vi "Average_center.vi"() -> ()   [LabVIEW 2012]
uses:
  <vilib>/Utility/file.llb/Read From Spreadsheet File (DBL).vi
  <vilib>/Analysis/baseanly.llb/Mean (DBL).vi
  <vilib>/Utility/file.llb/Write To Spreadsheet File (DBL).vi
  <vilib>/Analysis/NI_AALBase.lvlib
panel:
  out "mean":dbl format="%0.2f"
  in  "y shift":dbl
  in  "x shift":dbl
  in  "Write Data":bool
  out "XY Graph":cluster{dbl[], dbl[]}[](graph)
  in  "Group Fit":bool
  out "Array":dbl[][](array[numeric])
  out "last y":dbl
  out "last x":dbl
  out "last frame":dbl=30.0
  out "fit frame":dbl[](array[numeric])=[0.0, 0.0, 0.0, 0.0, 0.0, 0.0, 0.0, 0.0, 0.0, 0.0, 0.0, 0.0, 0.0, 0.0, 0.0, 0.0, 0.0, 0.0, 0.0, 0.0, 0.0, 0.0, 0.0, 0.0, 0.0, 0.0, 0.0, 0.0, 0.0, 0.0, 30.0, 31.0, 32.0, 33.0, 34.0, 35.0, 36.0, 37.0, 38.0, 39.0, 40.0, 41.0, 42.0, 43.0, 44.0, 45.0, 46.0, 47.0, 48.0, 49.0, 50.0, 51.0, 52.0, 53.0, 54.0, 55.0, 56.0, 57.0, 58.0, 59.0, 60.0, 61.0, 62.0, 63.0, 64.0, 65.0, 66.0, 67.0, 68.0, 69.0, 70.0, 71.0, 72.0, 73.0, 74.0, 75.0, 76.0, 77.0, 78.0, 79.0, 80.0, 81.0, 82.0, 83.0, 84.0, 85.0, 86.0, 87.0, 88.0, 89.0, 90.0, 91.0, 92.0, 93.0, 94.0, 95.0, 96.0, 97.0, 98.0, 99.0, 100.0, 101.0, 102.0, 103.0, 104.0, 105.0, 106.0, 107.0, 108.0, 109.0, 110.0, 111.0, 112.0, 113.0, 114.0, 115.0, 116.0, 117.0, 118.0, 119.0]
  out "Avg. in area":dbl
  out "Sub_region":dbl[][](graph)
  out "Masked region":dbl[][](graph)
  out "Mask":dbl[][](graph)
  in  "mask radius":dbl=15.0
  in  "Interp. multip.":i32=10
  out "subarray":u16[][](array[numeric])
  in  "sub region width":dbl=10.0
  out "y position":dbl[](array[numeric])
  out "x position":dbl[](array[numeric])
  out "Image Pixels (U16)":u16[][](graph)
  in  "Slide":i16(slide)=58 scale=0.0..109.0
  in  "stop":bool
  in  "Load Image":bool
  out "Array 3":u16[][][](array[numeric])
  out "all rows":dbl[][](array[numeric])=[[0.0, 0.0, 0.0, 0.0, 0.0, 0.0, 0.0, 0.0, 0.0, 0.0, 0.0, 0.0, 0.0, 0.0], [0.0, 0.0, 0.0, 0.0, 0.0, 0.0, 0.0, 0.0, 0.0, 0.0, 0.0, 0.0, 0.0, 0.0], [0.0, 0.0, 0.0, 0.0, 0.0, 0.0, 0.0, 0.0, 0.0, 0.0, 0.0, 0.0, 0.0, 0.0], [0.0, 0.0, 0.0, 0.0, 0.0, 0.0, 0.0, 0.0, 0.0, 0.0, 0.0, 0.0, 0.0, 0.0], [0.0, 0.0, 0.0, 0.0, 0.0, 0.0, 0.0, 0.0, 0.0, 0.0, 0.0, 0.0, 0.0, 0.0], [0.0, 0.0, 0.0, 0.0, 0.0, 0.0, 0.0, 0.0, 0.0, 0.0, 0.0, 0.0, 0.0, 0.0], [0.0, 0.0, 0.0, 0.0, 0.0, 0.0, 0.0, 0.0, 0.0, 0.0, 0.0, 0.0, 0.0, 0.0], [0.0, 0.0, 0.0, 0.0, 0.0, 0.0, 0.0, 0.0, 0.0, 0.0, 0.0, 0.0, 0.0, 0.0], [0.0, 0.0, 0.0, 0.0, 0.0, 0.0, 0.0, 0.0, 0.0, 0.0, 0.0, 0.0, 0.0, 0.0], [0.0, 0.0, 0.0, 0.0, 0.0, 0.0, 0.0, 0.0, 0.0, 0.0, 0.0, 0.0, 0.0, 0.0], [0.0, 0.0, 0.0, 0.0, 0.0, 0.0, 0.0, 0.0, 0.0, 0.0, 0.0, 0.0, 0.0, 0.0], [0.0, 0.0, 0.0, 0.0, 0.0, 0.0, 0.0, 0.0, 0.0, 0.0, 0.0, 0.0, 0.0, 0.0], [0.0, 0.0, 0.0, 0.0, 0.0, 0.0, 0.0, 0.0, 0.0, 0.0, 0.0, 0.0, 0.0, 0.0], [0.0, 0.0, 0.0, 0.0, 0.0, 0.0, 0.0, 0.0, 0.0, 0.0, 0.0, 0.0, 0.0, 0.0], [0.0, 0.0, 0.0, 0.0, 0.0, 0.0, 0.0, 0.0, 0.0, 0.0, 0.0, 0.0, 0.0, 0.0], [0.0, 0.0, 0.0, 0.0, 0.0, 0.0, 0.0, 0.0, 0.0, 0.0, 0.0, 0.0, 0.0, 0.0], [0.0, 0.0, 0.0, 0.0, 0.0, 0.0, 0.0, 0.0, 0.0, 0.0, 0.0, 0.0, 0.0, 0.0], [0.0, 0.0, 0.0, 0.0, 0.0, 0.0, 0.0, 0.0, 0.0, 0.0, 0.0, 0.0, 0.0, 0.0], [0.0, 0.0, 0.0, 0.0, 0.0, 0.0, 0.0, 0.0, 0.0, 0.0, 0.0, 0.0, 0.0, 0.0], [0.0, 0.0, 0.0, 0.0, 0.0, 0.0, 0.0, 0.0, 0.0, 0.0, 0.0, 0.0, 0.0, 0.0], [0.0, 0.0, 0.0, 0.0, 0.0, 0.0, 0.0, 0.0, 0.0, 0.0, 0.0, 0.0, 0.0, 0.0], [0.0, 0.0, 0.0, 0.0, 0.0, 0.0, 0.0, 0.0, 0.0, 0.0, 0.0, 0.0, 0.0, 0.0], [0.0, 0.0, 0.0, 0.0, 0.0, 0.0, 0.0, 0.0, 0.0, 0.0, 0.0, 0.0, 0.0, 0.0], [0.0, 0.0, 0.0, 0.0, 0.0, 0.0, 0.0, 0.0, 0.0, 0.0, 0.0, 0.0, 0.0, 0.0], [0.0, 0.0, 0.0, 0.0, 0.0, 0.0, 0.0, 0.0, 0.0, 0.0, 0.0, 0.0, 0.0, 0.0], [0.0, 0.0, 0.0, 0.0, 0.0, 0.0, 0.0, 0.0, 0.0, 0.0, 0.0, 0.0, 0.0, 0.0], [0.0, 0.0, 0.0, 0.0, 0.0, 0.0, 0.0, 0.0, 0.0, 0.0, 0.0, 0.0, 0.0, 0.0], [0.0, 0.0, 0.0, 0.0, 0.0, 0.0, 0.0, 0.0, 0.0, 0.0, 0.0, 0.0, 0.0, 0.0], [0.0, 0.0, 0.0, 0.0, 0.0, 0.0, 0.0, 0.0, 0.0, 0.0, 0.0, 0.0, 0.0, 0.0], [0.0, 0.0, 0.0, 0.0, 0.0, 0.0, 0.0, 0.0, 0.0, 0.0, 0.0, 0.0, 0.0, 0.0], [588.378, 571.636, 1951.749, 56.314, 30.0, 581.0, 565.0, 143.083, 56.314, 7.378, 6.636, 2.446, 2.255, 38.47], [588.991, 572.025, 2009.945, 50.246, 31.0, 582.0, 565.0, 140.68, 50.246, 6.991, 7.025, 2.63, 2.42, -21.441], [588.714, 571.844, 2675.103, 65.975, 32.0, 582.0, 565.0, 141.723, 65.975, 6.714, 6.844, 2.424, 2.662, -2.442], [588.923, 571.943, 2869.074, 59.276, 33.0, 582.0, 565.0, 141.386, 59.276, 6.923, 6.943, 3.108, 2.479, 16.634], [589.149, 572.219, 2964.71, 62.288, 34.0, 582.0, 565.0, 140.89, 62.288, 7.149, 7.219, 3.335, 2.272, 17.476], [589.117, 572.564, 3159.642, 76.028, 35.0, 582.0, 566.0, 142.616, 76.028, 7.117, 6.564, 2.391, 2.767, -34.678], [588.253, 571.858, 4815.994, 93.588, 36.0, 581.0, 565.0, 144.295, 93.588, 7.253, 6.858, 2.692, 3.042, -16.757], [588.57, 571.749, 4187.487, 108.1, 37.0, 582.0, 565.0, 138.967, 108.1, 6.57, 6.749, 2.497, 2.47, -4.575], [588.182, 571.554, 5165.682, 126.869, 38.0, 581.0, 565.0, 139.749, 126.869, 7.182, 6.554, 2.505, 2.587, -2.2], [588.137, 571.888, 4943.043, 129.295, 39.0, 581.0, 565.0, 140.974, 129.295, 7.137, 6.888, 2.405, 2.53, 47.476], [589.268, 572.233, 5097.999, 124.826, 40.0, 582.0, 565.0, 143.272, 124.826, 7.268, 7.233, 2.634, 2.467, 11.854], [589.304, 572.497, 5013.48, 120.72, 41.0, 582.0, 565.0, 143.383, 120.72, 7.304, 7.497, 2.698, 2.45, 49.572], [588.197, 572.522, 5839.616, 145.897, 42.0, 581.0, 566.0, 144.117, 145.897, 7.197, 6.522, 2.404, 2.65, 20.913], [589.318, 572.868, 5198.521, 138.498, 43.0, 582.0, 566.0, 148.006, 138.498, 7.318, 6.868, 2.36, 2.532, -41.707], [589.3, 573.241, 5837.78, 129.56, 44.0, 582.0, 566.0, 145.37, 129.56, 7.3, 7.241, 2.489, 2.881, -15.221], [589.227, 572.842, 5580.823, 129.117, 45.0, 582.0, 566.0, 141.209, 129.117, 7.227, 6.842, 2.535, 2.714, -41.207], [588.149, 572.449, 5701.334, 142.324, 46.0, 581.0, 565.0, 143.335, 142.324, 7.149, 7.449, 2.454, 2.598, -32.721], [589.384, 572.935, 6227.49, 151.874, 47.0, 582.0, 566.0, 141.157, 151.874, 7.384, 6.935, 2.598, 2.512, 19.737], [589.449, 572.711, 5978.315, 137.65, 48.0, 582.0, 566.0, 143.017, 137.65, 7.449, 6.711, 2.735, 2.528, 8.159], [589.244, 572.624, 5919.357, 148.112, 49.0, 582.0, 566.0, 142.639, 148.112, 7.244, 6.624, 2.58, 2.465, -12.336], [588.598, 572.304, 6268.99, 145.526, 50.0, 582.0, 565.0, 141.281, 145.526, 6.598, 7.304, 2.701, 2.538, 33.088], [588.846, 571.332, 6648.118, 161.592, 51.0, 582.0, 564.0, 144.772, 161.592, 6.846, 7.332, 2.526, 2.592, -35.807], [588.275, 571.664, 6807.061, 156.088, 52.0, 581.0, 565.0, 141.756, 156.088, 7.275, 6.664, 2.582, 2.688, -11.2], [589.294, 571.895, 7384.551, 170.132, 53.0, 582.0, 565.0, 143.89, 170.132, 7.294, 6.895, 2.756, 2.507, 0.831], [589.111, 571.679, 6844.837, 168.548, 54.0, 582.0, 565.0, 146.967, 168.548, 7.111, 6.679, 2.608, 2.479, 35.063], [588.084, 572.968, 8218.547, 186.106, 55.0, 581.0, 566.0, 143.954, 186.106, 7.084, 6.968, 2.57, 2.734, -19.232], [587.815, 572.729, 7363.057, 172.996, 56.0, 581.0, 566.0, 147.824, 172.996, 6.815, 6.729, 2.546, 2.661, -17.096], [588.099, 572.865, 7172.664, 169.509, 57.0, 581.0, 566.0, 146.475, 169.509, 7.099, 6.865, 2.529, 2.662, 3.276], [588.613, 573.319, 7735.74, 168.13, 58.0, 582.0, 566.0, 143.465, 168.13, 6.613, 7.319, 2.731, 2.682, -41.964], [589.311, 571.883, 8510.861, 175.523, 59.0, 582.0, 565.0, 146.987, 175.523, 7.311, 6.883, 2.954, 2.613, -6.69], [589.618, 573.49, 7491.265, 171.756, 60.0, 583.0, 566.0, 144.839, 171.756, 6.618, 7.49, 2.541, 2.732, -31.862], [589.911, 572.603, 7668.811, 181.544, 61.0, 583.0, 566.0, 146.029, 181.544, 6.911, 6.603, 2.513, 2.675, -30.525], [589.501, 571.738, 7956.749, 183.055, 62.0, 583.0, 565.0, 145.504, 183.055, 6.501, 6.738, 2.586, 2.675, -41.477], [588.621, 573.102, 6517.135, 165.088, 63.0, 582.0, 566.0, 144.24, 165.088, 6.621, 7.102, 2.55, 2.464, 30.68], [588.614, 572.262, 8097.09, 188.474, 64.0, 582.0, 565.0, 148.629, 188.474, 6.614, 7.262, 2.684, 2.547, 21.023], [588.412, 573.225, 7667.721, 187.156, 65.0, 581.0, 566.0, 146.037, 187.156, 7.412, 7.225, 2.533, 2.574, -14.326], [589.138, 572.17, 7419.61, 187.712, 66.0, 582.0, 565.0, 144.966, 187.712, 7.138, 7.17, 2.439, 2.579, 2.576], [588.447, 573.003, 7447.27, 184.552, 67.0, 581.0, 566.0, 144.056, 184.552, 7.447, 7.003, 2.482, 2.588, -20.753], [588.797, 572.666, 7931.613, 194.41, 68.0, 582.0, 566.0, 152.26, 194.41, 6.797, 6.666, 2.482, 2.616, -40.942], [589.035, 573.273, 7506.722, 176.286, 69.0, 582.0, 566.0, 151.999, 176.286, 7.035, 7.273, 2.56, 2.647, -3.932], [589.161, 573.188, 7064.163, 164.387, 70.0, 582.0, 566.0, 146.684, 164.387, 7.161, 7.188, 2.491, 2.746, -35.275], [589.179, 572.692, 8239.039, 198.212, 71.0, 582.0, 566.0, 145.03, 198.212, 7.179, 6.692, 2.52, 2.625, -45.273], [589.244, 573.071, 7797.946, 184.243, 72.0, 582.0, 566.0, 143.867, 184.243, 7.244, 7.071, 2.531, 2.662, -24.69], [589.224, 572.754, 8253.451, 190.47, 73.0, 582.0, 566.0, 147.41, 190.47, 7.224, 6.754, 2.688, 2.566, -44.285], [589.246, 573.147, 8317.649, 190.611, 74.0, 582.0, 566.0, 146.642, 190.611, 7.246, 7.147, 2.55, 2.723, -32.822], [589.752, 572.947, 9105.262, 213.77, 75.0, 583.0, 566.0, 147.127, 213.77, 6.752, 6.947, 2.662, 2.547, 32.368], [589.3, 572.52, 7862.343, 187.84, 76.0, 582.0, 566.0, 149.161, 187.84, 7.3, 6.52, 2.662, 2.503, 29.332], [589.204, 572.969, 8335.052, 189.604, 77.0, 582.0, 566.0, 151.964, 189.604, 7.204, 6.969, 2.717, 2.575, 58.933], [589.499, 572.757, 9006.146, 198.994, 78.0, 583.0, 566.0, 149.984, 198.994, 6.499, 6.757, 2.752, 2.618, 32.907], [589.397, 572.902, 7734.161, 193.866, 79.0, 582.0, 566.0, 145.231, 193.866, 7.397, 6.902, 2.486, 2.554, -27.493], [589.693, 573.01, 8179.008, 185.925, 80.0, 583.0, 566.0, 140.741, 185.925, 6.693, 7.01, 2.707, 2.586, 35.872], [589.822, 572.721, 8146.537, 187.516, 81.0, 583.0, 566.0, 142.557, 187.516, 6.822, 6.721, 2.709, 2.552, 24.18], [590.124, 573.067, 8304.198, 206.646, 82.0, 583.0, 566.0, 148.363, 206.646, 7.124, 7.067, 2.541, 2.517, 8.341], [589.729, 572.752, 8814.258, 196.005, 83.0, 583.0, 566.0, 144.289, 196.005, 6.729, 6.752, 2.606, 2.747, -26.134], [590.29, 572.188, 9195.381, 211.579, 84.0, 583.0, 565.0, 152.314, 211.579, 7.29, 7.188, 2.554, 2.708, -43.327], [589.688, 572.894, 8639.23, 193.751, 85.0, 583.0, 566.0, 150.623, 193.751, 6.688, 6.894, 2.651, 2.677, -1.432], [590.354, 572.918, 8226.652, 199.952, 86.0, 583.0, 566.0, 157.956, 199.952, 7.354, 6.918, 2.492, 2.628, -25.03], [590.029, 572.212, 9007.563, 213.549, 87.0, 583.0, 565.0, 160.746, 213.549, 7.029, 7.212, 2.612, 2.57, 26.402], [590.667, 572.953, 8180.464, 189.378, 88.0, 584.0, 566.0, 163.384, 189.378, 6.667, 6.953, 2.504, 2.745, -28.032], [590.214, 572.86, 9370.796, 202.878, 89.0, 583.0, 566.0, 165.841, 202.878, 7.214, 6.86, 2.809, 2.617, -4.851], [590.209, 572.642, 9321.677, 192.963, 90.0, 583.0, 566.0, 167.56, 192.963, 7.209, 6.642, 2.827, 2.72, 26.973], [590.106, 572.819, 8578.763, 187.192, 91.0, 583.0, 566.0, 167.636, 187.192, 7.106, 6.819, 2.764, 2.639, 0.733], [589.109, 572.606, 9199.084, 205.973, 92.0, 582.0, 566.0, 170.548, 205.973, 7.109, 6.606, 2.839, 2.504, -26.634], [589.621, 573.464, 8713.76, 199.642, 93.0, 583.0, 566.0, 173.91, 199.642, 6.621, 7.464, 2.578, 2.695, 20.491], [589.416, 572.96, 9245.449, 192.478, 94.0, 582.0, 566.0, 168.759, 192.478, 7.416, 6.96, 2.846, 2.686, 18.797], [589.287, 573.811, 8898.641, 205.443, 95.0, 582.0, 567.0, 165.694, 205.443, 7.287, 6.811, 2.565, 2.688, -25.953], [589.75, 574.063, 8666.373, 194.701, 96.0, 583.0, 567.0, 162.51, 194.701, 6.75, 7.063, 2.628, 2.696, 57.72], [589.228, 573.563, 7372.072, 165.971, 97.0, 582.0, 567.0, 168.454, 165.971, 7.228, 6.563, 2.592, 2.728, -23.62], [589.331, 573.587, 7472.889, 171.395, 98.0, 582.0, 567.0, 164.698, 171.395, 7.331, 6.587, 2.708, 2.562, 28.535], [589.511, 573.832, 7166.854, 162.98, 99.0, 583.0, 567.0, 163.229, 162.98, 6.511, 6.832, 2.578, 2.715, -20.163], [589.682, 573.682, 6816.553, 154.245, 100.0, 583.0, 567.0, 165.097, 154.245, 6.682, 6.682, 2.589, 2.717, -21.174], [589.486, 573.735, 6823.353, 153.239, 101.0, 582.0, 567.0, 166.149, 153.239, 7.486, 6.735, 2.769, 2.559, 40.663], [589.345, 574.012, 5916.487, 145.218, 102.0, 582.0, 567.0, 166.02, 145.218, 7.345, 7.012, 2.459, 2.637, -29.362], [589.596, 573.28, 7035.411, 162.246, 103.0, 583.0, 566.0, 168.688, 162.246, 6.596, 7.28, 2.701, 2.555, 13.303], [590.31, 573.435, 7161.38, 154.707, 104.0, 583.0, 566.0, 167.669, 154.707, 7.31, 7.435, 2.596, 2.838, -36.495], [589.783, 572.85, 6720.292, 156.126, 105.0, 583.0, 566.0, 166.76, 156.126, 6.783, 6.85, 2.749, 2.492, 24.548], [591.015, 572.749, 7014.993, 157.259, 106.0, 584.0, 566.0, 165.394, 157.259, 7.015, 6.749, 2.562, 2.772, 41.853], [590.243, 572.657, 6684.99, 139.06, 107.0, 583.0, 566.0, 170.161, 139.06, 7.243, 6.657, 2.68, 2.855, -27.177], [590.097, 572.626, 6605.271, 147.395, 108.0, 583.0, 566.0, 167.235, 147.395, 7.097, 6.626, 2.584, 2.76, -46.676], [589.755, 572.962, 6684.835, 150.619, 109.0, 583.0, 566.0, 168.965, 150.619, 6.755, 6.962, 2.588, 2.73, -43.616], [590.045, 573.678, 7248.207, 157.593, 110.0, 583.0, 567.0, 169.026, 157.593, 7.045, 6.678, 2.755, 2.657, -27.85], [589.882, 572.915, 6522.802, 161.728, 111.0, 583.0, 566.0, 168.486, 161.728, 6.882, 6.915, 2.586, 2.482, 39.242], [589.936, 573.137, 7469.372, 160.636, 112.0, 583.0, 566.0, 169.026, 160.636, 6.936, 7.137, 2.749, 2.692, 27.624], [589.945, 573.049, 6553.532, 149.638, 113.0, 583.0, 566.0, 172.505, 149.638, 6.945, 7.049, 2.567, 2.715, -20.849], [589.842, 573.25, 6651.382, 154.162, 114.0, 583.0, 566.0, 170.271, 154.162, 6.842, 7.25, 2.511, 2.735, -29.909], [589.791, 573.291, 7647.773, 151.64, 115.0, 583.0, 566.0, 167.938, 151.64, 6.791, 7.291, 2.739, 2.93, -32.783], [590.391, 572.528, 7485.002, 167.83, 116.0, 583.0, 566.0, 169.628, 167.83, 7.391, 6.528, 2.647, 2.682, -63.794], [591.156, 573.249, 6252.507, 151.093, 117.0, 584.0, 566.0, 171.68, 151.093, 7.156, 7.249, 2.463, 2.674, -32.952], [590.608, 572.969, 6267.337, 151.056, 118.0, 584.0, 566.0, 169.338, 151.056, 6.608, 6.969, 2.493, 2.649, -31.422], [590.835, 573.768, 5979.319, 136.177, 119.0, 584.0, 567.0, 165.497, 136.177, 6.835, 6.768, 2.565, 2.725, -30.434]] format="%0.3f"
  in  "Spreadsheet":path
  in  "Inverse Image?":bool
  in  "Flip Width/Length?":bool=TRUE
  in  "Data in IFD\n(small files)":bool=TRUE
  in  "File Path image":path
  # "Shift averaging relative to fit"
  # "This sofware takes a .tiff stack and x,y position of a fit puncta to find the average intensity of a masked region.  Interpolation is done to get subpixel region for mask."
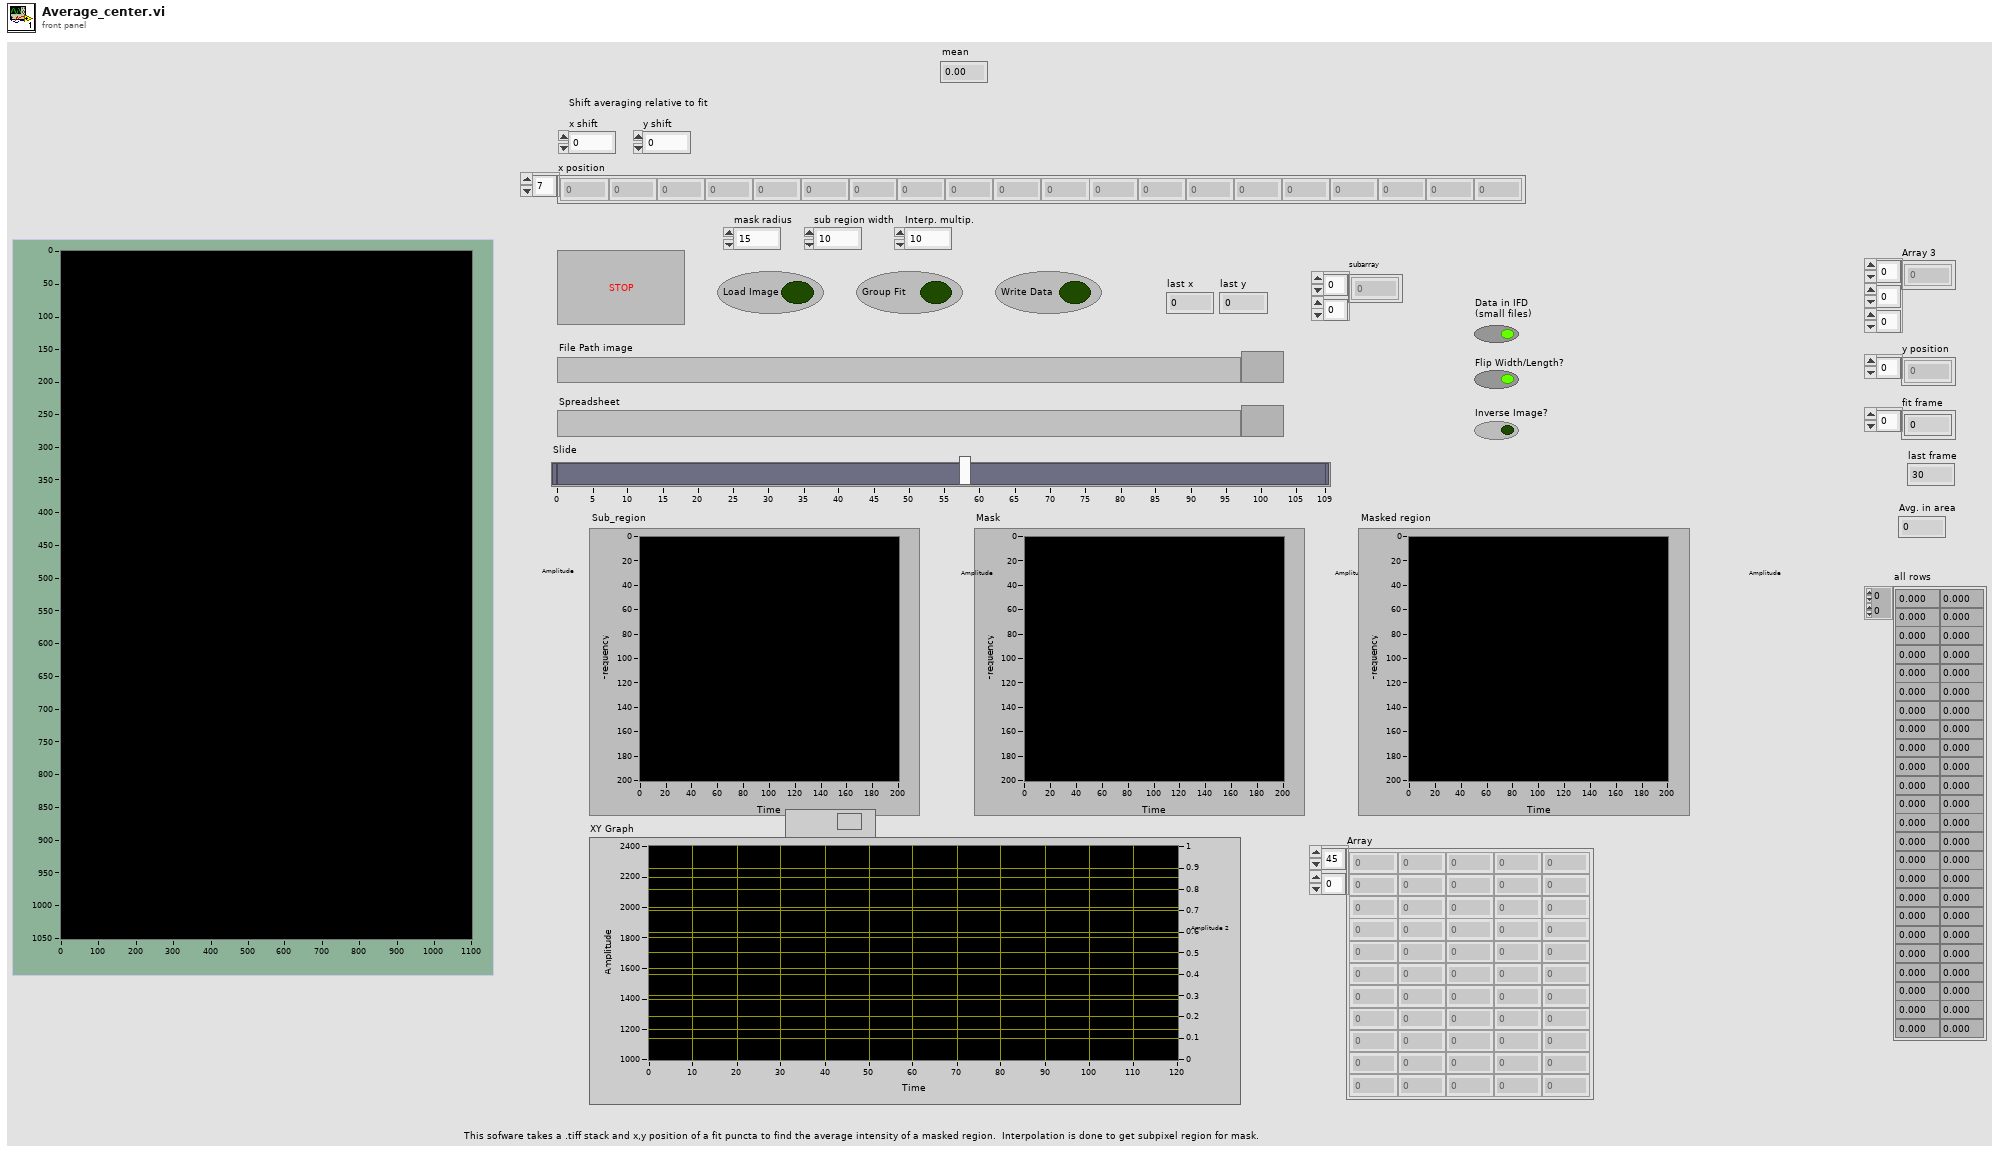
[diagram p1: front panel]
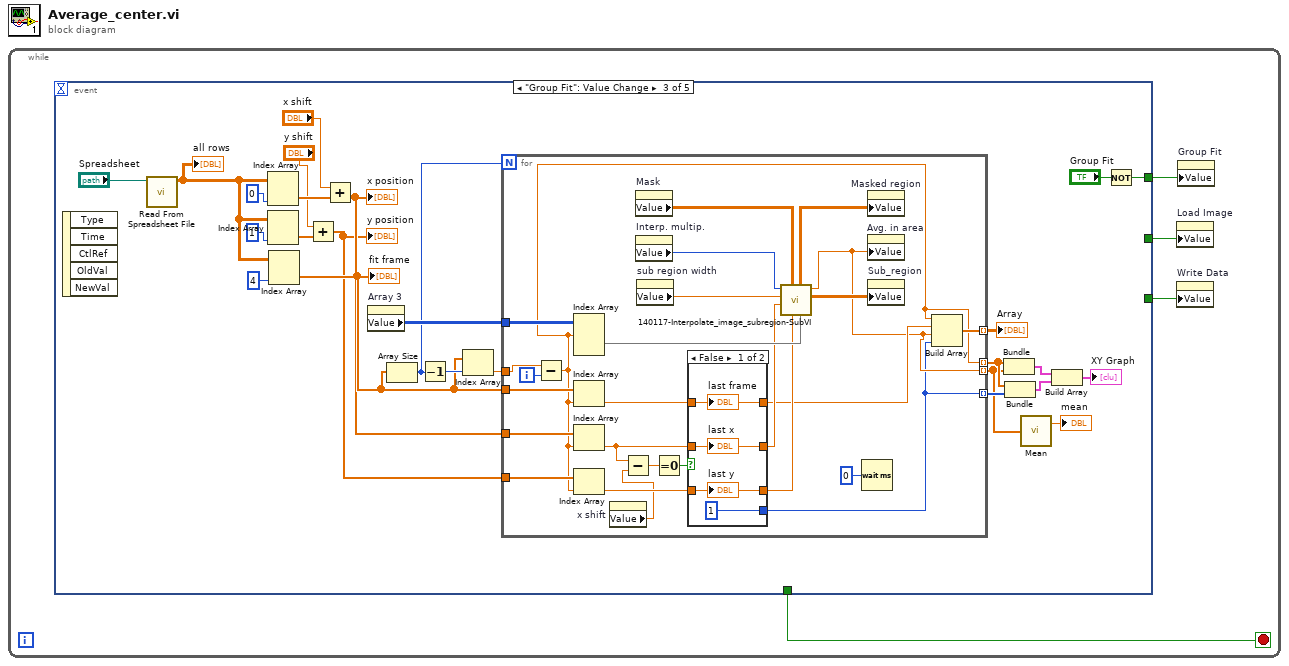
[diagram p0: block diagram]
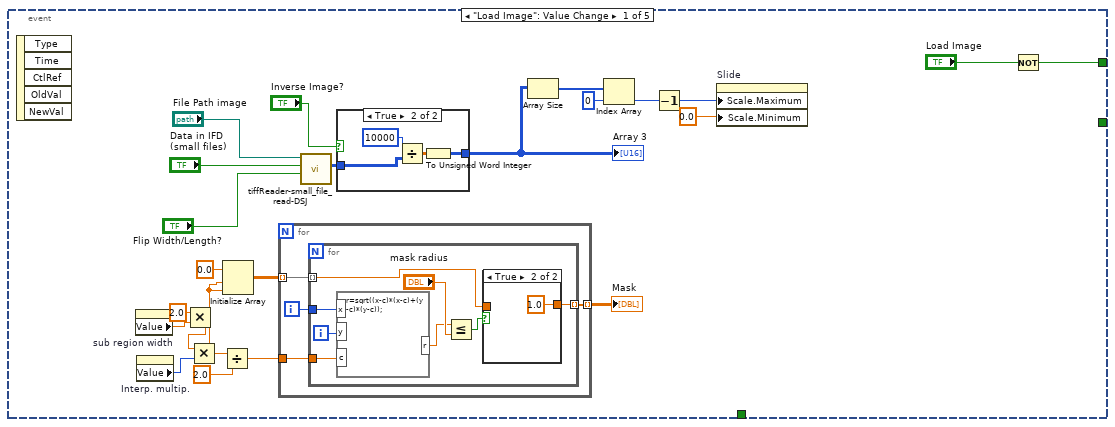
[diagram p2: hidden frame]
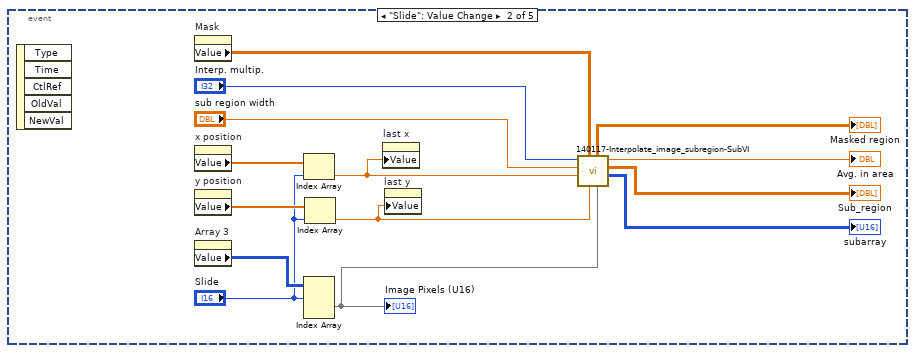
[diagram p5: hidden frame]
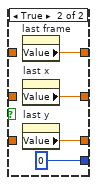
[diagram p6: hidden frame]
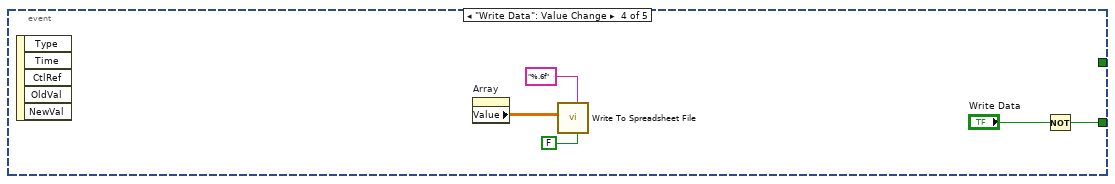
[diagram p7: hidden frame]
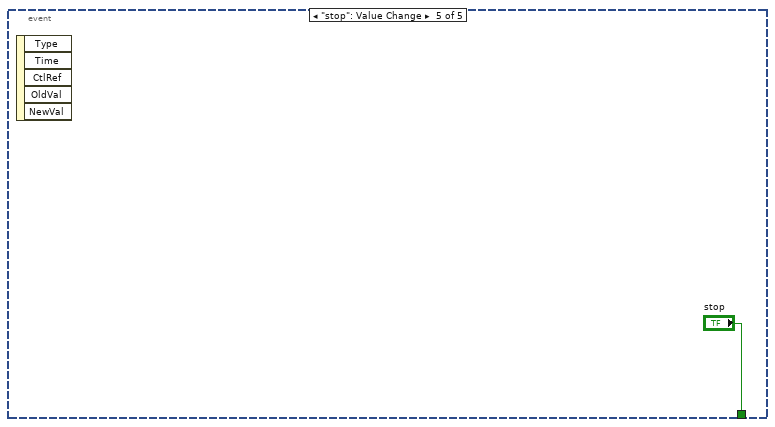
[diagram p8: hidden frame]
diagram:
  n1 = while {
    stop <- w3 stop-if-true
    n2 = event shown="[2] \"Group Fit\": Value Change" {
      selector: _ -> [_ _ _ _ _]
      dyn-events: _ -> [_ _ _ _ _]
      timeout: _ -> [_ _ _ _ _]
      tunnel: [w21 _ _ _ _] -> w4
      tunnel: [_ _ _ _ "stop"] -> w3
      tunnel: [_ _ w80 _ _] -> w2
      tunnel: [_ _ _ w122 _] -> w1
      event "Load Image": Value Change {
        n3 = event-data() -> ()  [unwired: 1 in, 5 out]
        n4 = property on="sub region width" class="DigNum (strict)"() -> ("Value"=w7:dbl)  [unwired: 2 in, 2 out]
        n5 = property on="Interp. multip." class="DigNum (strict)"() -> ("Value"=w13:i32)  [unwired: 2 in, 2 out]
        n6 = Multiply(x=2.0, y=w7) -> (x*y=w6:dbl)
        n7 = Multiply(x=w6, y=w13) -> (x*y=w11:dbl)
        n8 = Divide(x=w11, y=2.0) -> (x/y=w9:dbl)
        n9 = Initialize Array(0.0 ("element"), w11, w11) -> (w12:dbl[][])
        n10 = for {
          tunnel: w12 -> [w31] mode=indexing
          tunnel: w9 -> [w30]
          tunnel: [w28] -> w8 mode=indexing
          i -> [w29]
          n11 = for {
            tunnel: w31 -> [w35] mode=indexing
            tunnel: w30 -> [w39]
            tunnel: w29 -> [w38]
            tunnel: [w34] -> w28 mode=indexing
            i -> [w37]
            n12 = formula code="r=sqrt((x-c)*(x-c)+(y-c)*(y-c));"("x"=w38, "c"=w39, "y"=w37) -> ("r"=w32:dbl)
            n13 = Less Or Equal?(x=w32, y="mask radius") -> (x <= y?=w36:bool)
            n14 = case shown="True" w36 {
              tunnel: w35 -> [w40 _]
              tunnel: [w40 1.0 ("element")] -> w34
              frame False {
              }
              frame True {
              }
            }
          }
        }
        "Mask" <- w8
        n15 = call "tiffReader-small_file_read-DSJ.vi"("Flip Width/Length?"="Flip Width/Length?", "Data in IFD\n(small files)"="Data in IFD\n(small files)", "File Path"="File Path image") -> ("Array 3"=w24:u16[][][])  [unwired: 1 in, 3 out]
        n16 = case shown="True" "Inverse Image?" {
          tunnel: w24 -> [w42 w46]
          tunnel: [w42 w43] -> w15
          frame False {
          }
          frame True {
            n17 = Divide(x=10000 ("dimension size"), y=w46) -> (x/y=w44:dbl[][][])
            n18 = To Unsigned Word Integer(number=w44) -> (unsigned 16bit integer=w43:u16[][][])
          }
        }
        "Array 3" <- w15
        n19 = Array Size(array=w15) -> (size(s)=w18:i32[])
        n20 = Index Array(array=w18, index=0) -> (element=w20:i32)
        n21 = Decrement(x=w20) -> (x-1=w16:i32)
        n22 = property on="Slide" class="Slide (strict)"("Scale.Maximum"=w16, "Scale.Minimum"=0.0 ("Scale.Range:Minimum")) -> ()  [unwired: 2 in, 2 out]
        n23 = Not(x="Load Image") -> (.not. x?=w21:bool)
      }
      event "Slide": Value Change {
        n24 = event-data() -> ()  [unwired: 1 in, 5 out]
        n25 = property on="Mask" class="IntGraph (strict)"() -> ("Value"=w50:dbl[][])  [unwired: 2 in, 2 out]
        n26 = property on="x position" class="Arr (strict)"() -> ("Value"=w58:dbl[])  [unwired: 2 in, 2 out]
        n27 = property on="y position" class="Arr (strict)"() -> ("Value"=w57:dbl[])  [unwired: 2 in, 2 out]
        n28 = property on="Array 3" class="Arr (strict)"() -> ("Value"=w60:u16[][][])  [unwired: 2 in, 2 out]
        n29 = Index Array(array=w58, index="Slide") -> (element=w49:dbl)
        n30 = Index Array(array=w60, index (dim 0)="Slide") -> (element=w56:u16[][])  [unwired: 2 in]
        "Image Pixels (U16)" <- w56
        n31 = Index Array(array=w57, index="Slide") -> (element=w48:dbl)
        n32 = property on="last x" class="DigNum (strict)"("Value"=w49) -> ()  [unwired: 2 in, 2 out]
        n33 = property on="last y" class="DigNum (strict)"("Value"=w48) -> ()  [unwired: 2 in, 2 out]
        n34 = call "140117-Interpolate_image_subregion-SubVI.vi"("Image"=w56, "y fit position"=w48, "Mask"=w50, "x fit position"=w49, "sub region width"="sub region width", "Interp. multip."="Interp. multip.") -> ("Sub Image"=→"subarray":u16[][], "Array"=→"Sub_region":dbl[][], "Avg. in area"=→"Avg. in area":dbl, "Masked region"=→"Masked region":dbl[][])  [unwired: 2 in]
      }
      event "Group Fit": Value Change {
        n35 = event-data() -> ()  [unwired: 1 in, 5 out]
        n36 = call-poly <vilib>:"Read From Spreadsheet File.vi"("file path (dialog if empty)"="Spreadsheet") -> ("all rows"=w71:dbl[][])  [unwired: 6 in, 4 out]
        "all rows" <- w71
        n37 = Index Array(array=w71, index (col)=0 ("index (row)")) -> (element=w67:dbl[])  [unwired: 1 in]
        n38 = Index Array(array=w71, index (col)=1 ("index (row)")) -> (element=w65:dbl[])  [unwired: 1 in]
        n39 = Index Array(array=w71, index (col)=4 ("disabled index (col)")) -> (element=w69:dbl[])  [unwired: 1 in]
        "fit frame" <- w69
        n40 = Add(x="y shift", y=w65) -> (x+y=w64:dbl[])
        "y position" <- w64
        n41 = Add(x="x shift", y=w67) -> (x+y=w66:dbl[])
        "x position" <- w66
        n42 = property on="Array 3" class="Arr (strict)"() -> ("Value"=w86:u16[][][])  [unwired: 2 in, 2 out]
        n43 = Array Size(array=w69) -> (size(s)=w82:i32)
        n44 = Decrement(x=w82) -> (x-1=w85:i32)
        n45 = Index Array(array=w69, index=w85) -> (element=w84:dbl)
        n46 = for {
          N: w82 -> [_]
          tunnel: w86 -> [w105]
          tunnel: w69 -> [w112]
          tunnel: w66 -> [w110]
          tunnel: w64 -> [w109]
          tunnel: w84 -> [w111]
          tunnel: [w95] -> w83 mode=indexing
          tunnel: [w92] -> w79 mode=indexing
          tunnel: [w91] -> w62 mode=indexing
          tunnel: [w90] -> w78 mode=indexing
          i -> [w94]
          n47 = Subtract(x=w111, y=w94) -> (x-y=w92:dbl)
          n48 = Index Array(array=w105, index (dim 0)=w92) -> (element=w104:u16[][])  [unwired: 2 in]
          n49 = Index Array(array=w112, index=w92) -> (element=w107:dbl)
          n50 = Index Array(array=w110, index=w92) -> (element=w89:dbl)
          n51 = Index Array(array=w109, index=w92) -> (element=w106:dbl)
          n52 = property on="x shift" class="DigNum (strict)"() -> ("Value"=w87:dbl)  [unwired: 2 in, 2 out]
          n53 = Subtract(x=w89, y=w87) -> (x-y=w88:dbl)
          n54 = property on="Mask" class="IntGraph (strict)"() -> ("Value"=w99:dbl[][])  [unwired: 2 in, 2 out]
          n55 = property on="Interp. multip." class="DigNum (strict)"() -> ("Value"=w100:i32)  [unwired: 2 in, 2 out]
          n56 = property on="sub region width" class="DigNum (strict)"() -> ("Value"=w101:dbl)  [unwired: 2 in, 2 out]
          n57 = Equal To 0?(x=w88) -> (x = 0?=w108:bool)
          n58 = case shown="False" w108 {
            tunnel: w107 -> [w116 _]
            tunnel: w106 -> [w113 _]
            tunnel: w89 -> [w114 _]
            tunnel: [w116 w118] -> w96
            tunnel: [w114 w120] -> w102
            tunnel: [w113 w119] -> w103
            tunnel: [1 0] -> w90
            frame False {
              "last frame" <- w116
              "last x" <- w114
              "last y" <- w113
            }
            frame True {
              n59 = property on="last frame" class="DigNum (strict)"() -> ("Value"=w118:dbl)  [unwired: 2 in, 2 out]
              n60 = property on="last x" class="DigNum (strict)"() -> ("Value"=w120:dbl)  [unwired: 2 in, 2 out]
              n61 = property on="last y" class="DigNum (strict)"() -> ("Value"=w119:dbl)  [unwired: 2 in, 2 out]
            }
          }
          n62 = call "140117-Interpolate_image_subregion-SubVI.vi"("Image"=w104, "y fit position"=w103, "Mask"=w99, "x fit position"=w102, "sub region width"=w101, "Interp. multip."=w100) -> ("Array"=w97:dbl[][], "Avg. in area"=w91:dbl, "Masked region"=w98:dbl[][])  [unwired: 2 in, 1 out]
          n63 = Wait (ms)(milliseconds to wait=u32 0) -> ()  [unwired: 1 out]
          n64 = property on="Masked region" class="IntGraph (strict)"("Value"=w98) -> ()  [unwired: 2 in, 2 out]
          n65 = property on="Avg. in area" class="DigNum (strict)"("Value"=w91) -> ()  [unwired: 2 in, 2 out]
          n66 = property on="Sub_region" class="IntGraph (strict)"("Value"=w97) -> ()  [unwired: 2 in, 2 out]
          n67 = Build Array(w92, w96, w91, w90) -> (w95:dbl[])
        }
        "Array" <- w83
        n68 = Bundle(w79, w62) -> (w76:cluster{dbl[], dbl[]})  [unwired: 1 in]
        n69 = Bundle(w79, w78) -> (w77:cluster{dbl[], i32[]})  [unwired: 1 in]
        n70 = call-poly <vilib>:"Mean.vi"("X"=w62) -> ("mean"=→"mean":dbl)  [unwired: 1 out]
        n71 = Build Array(w76, w77) -> (→"XY Graph":cluster{dbl[], dbl[]}[])
        n72 = Not(x="Group Fit") -> (.not. x?=w80:bool)
      }
      event "Write Data": Value Change {
        n73 = event-data() -> ()  [unwired: 1 in, 5 out]
        n74 = property on="Array" class="Arr (strict)"() -> ("Value"=w125:dbl[][])  [unwired: 2 in, 2 out]
        n75 = call-poly <vilib>:"Write To Spreadsheet File.vi"("transpose? (no:F)"=FALSE, "format (%.3f)"="%.6f", "2D data"=w125) -> ()  [unwired: 5 in, 1 out]
        n76 = Not(x="Write Data") -> (.not. x?=w122:bool)
      }
      event "stop": Value Change {
        n77 = event-data() -> ()  [unwired: 1 in, 5 out]
      }
    }
    n78 = property on="Load Image" class="Bool (strict)"("Value"=w4) -> ()  [unwired: 2 in, 2 out]
    n79 = property on="Write Data" class="Bool (strict)"("Value"=w1) -> ()  [unwired: 2 in, 2 out]
    n80 = property on="Group Fit" class="Bool (strict)"("Value"=w2) -> ()  [unwired: 2 in, 2 out]
  }
